vi "PDCGetAllStates.vi"(8 "error in (no error)":errorcluster, 10 "PDCLists":T5, 11 "PDCAllStates in":T1={"DeviceNo"=0, "ChildNo"=1, "ColorType"=enum."MONO", "BitDepth"=0, "Resolution"={"Width"=0, "Height"=0}, "RecordRate"=0, "ShutterSpeed"=0, "TriggerMode"=0, "Display"=enum."LiveStop", "PDCRecordStatus"=enum."Live", "PlayFrames"=FALSE, "Start Frame"=0, "Current Frame"=0, "End Frame"=0, "RefImage8bit"=[], "RefImage16bit"=[], "Auto Trigger"=FALSE, "PDCSettings"={"Interface"=enum."Gigabit-Ethernet", "AutoSearch"=FALSE, "IP - AutoSearch"=[], "IP - Direct"=[], "Simulate"=FALSE}}) -> (0 "error out":errorcluster, 2 "PDC Setup":T6={"Color Type"=enum."MONO", "Bit Depth"=0, "Resolution"=0, "Record Rate"=0, "Shutter Speed"=0, "Trigger Mode"=0, "Display"=enum."LiveStop"} {"Trigger Mode" items=["START", "CENTER", "END", "MANUAL", "RANDOM", "RANDOM_RESET", "RANDOM_CENTER", "RANDOM_MANUAL", "START", "START"]; "Shutter Speed" items=["1/42772 sec", "1/44444 sec", "1/47058 sec", "1/50000 sec", "1/53333 sec", "1/57142 sec", "1/61538 sec", "1/66666 sec", "1/72727 sec", "1/80000 sec", "1/88888 sec", "1/100000 sec", "1/114285 sec", "1/133333 sec", "1/160000 sec", "1/200000 sec", "1/266666 sec", "1/400000 sec", "1/800000 sec", "1/996923 sec", "1/1246154 sec", "1/1661538 sec", "1/2700000 sec", "1/3410526 sec"]; "Resolution" items=["768 X 416", "896 X 368", "768 X 328", "768 X 272", "640 X 256", "512 X 512", "512 X 272", "512 X 256", "384 X 264", "256 X 256", "256 X 152", "256 X 128", "256 X 80", "128 X 128", "128 X 48", "128 X 40", "128 X 16", "128 X 8"]; "Record Rate" items=["50 fps", "60 fps", "125 fps", "250 fps", "500 fps", "1000 fps", "2000 fps", "3000 fps", "4000 fps", "5000 fps", "6000 fps", "7200 fps", "8000 fps", "9000 fps", "10000 fps", "12500 fps", "13500 fps", "20000 fps", "30000 fps", "40000 fps", "50000 fps", "60000 fps", "72000 fps", "81000 fps", "100000 fps", "200000 fps", "300000 fps", "480000 fps", "540000 fps", "675000 fps", "900000 fps", "1080000 fps"]}, 3 "PDCAllStates out":T1={"DeviceNo"=0, "ChildNo"=1, "ColorType"=enum."MONO", "BitDepth"=0, "Resolution"={"Width"=0, "Height"=0}, "RecordRate"=0, "ShutterSpeed"=0, "TriggerMode"=0, "Display"=enum."LiveStop", "PDCRecordStatus"=enum."Live", "PlayFrames"=FALSE, "Start Frame"=0, "Current Frame"=0, "End Frame"=0, "RefImage8bit"=[], "RefImage16bit"=[], "Auto Trigger"=FALSE, "PDCSettings"={"Interface"=enum."Gigabit-Ethernet", "AutoSearch"=FALSE, "IP - AutoSearch"=[], "IP - Direct"=[], "Simulate"=FALSE}})   [LabVIEW 2015]
uses:
  TypeDefs/PDCSetup.ctl
  TypeDefs/PDCDisplay.ctl
  TypeDefs/PDCAllStates.ctl
  TypeDefs/PDCRecordStatus.ctl
  TypeDefs/PDCSettings.ctl
  TypeDefs/PDCLists.ctl
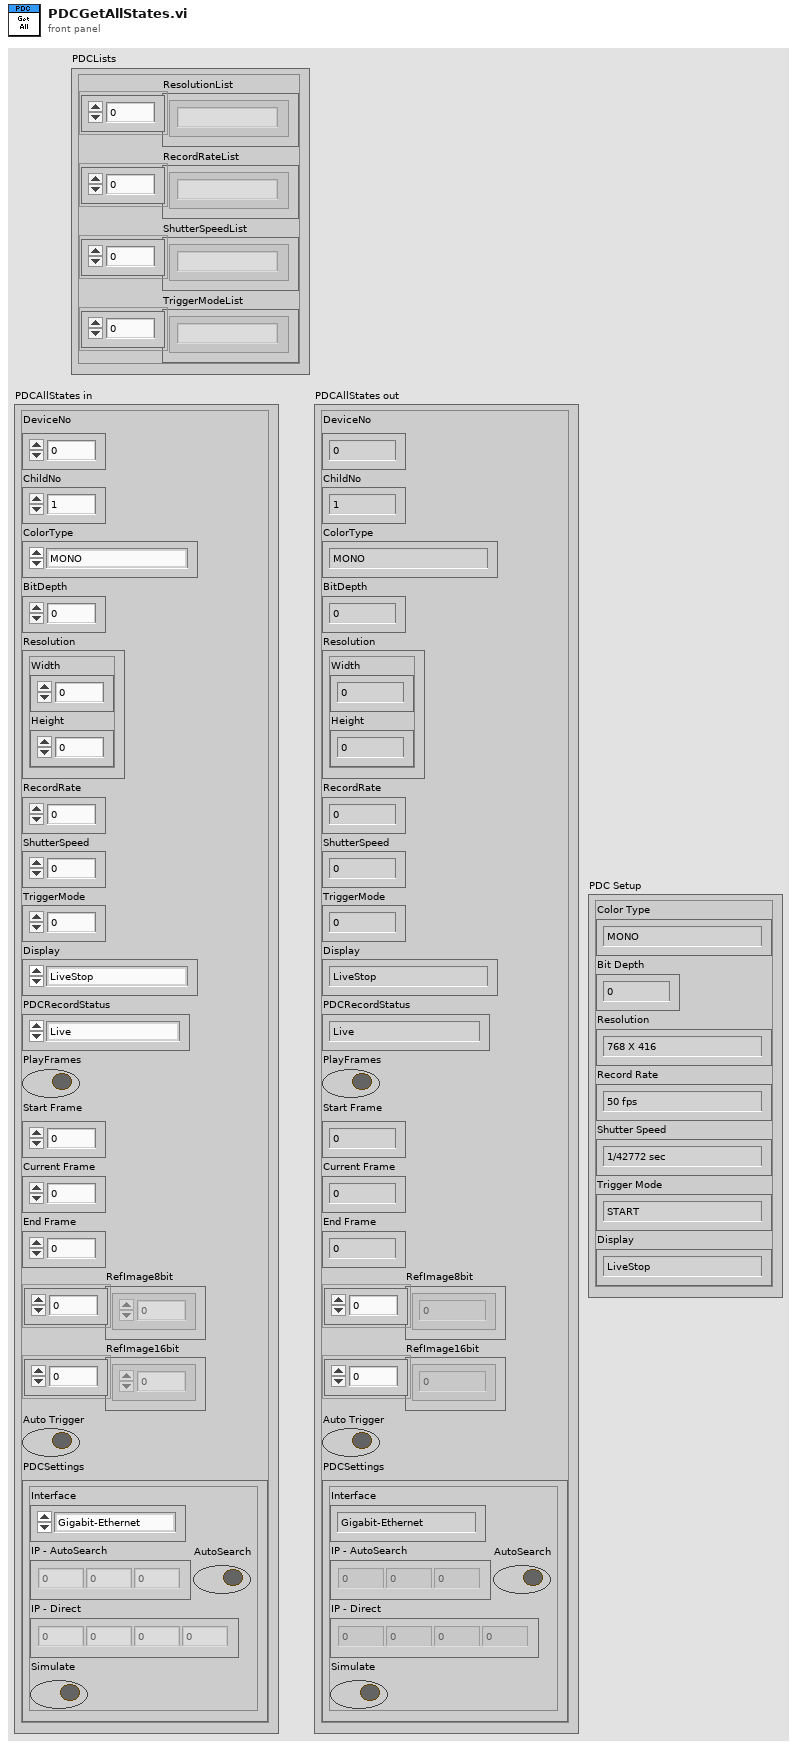
[diagram p1: front panel]
types:
  T1 = typedef "PDCAllStates.ctl" = cluster{"DeviceNo":u32, "ChildNo":u32, "ColorType":enum16{"MONO", "COLOR"}, "BitDepth":i8, "Resolution":cluster{"Width":u32, "Height":u32}, "RecordRate":u32, "ShutterSpeed":u32, "TriggerMode":u32, "Display":T2, "PDCRecordStatus":T3, "PlayFrames":bool, "Start Frame":i32, "Current Frame":i32, "End Frame":i32, "RefImage8bit":u8[], "RefImage16bit":u16[], "Auto Trigger":bool, "PDCSettings":T4}
  T2 = typedef "PDCDisplay.ctl" = enum16{"Live", "Memory", "LiveStop"}
  T3 = typedef "PDCRecordStatus.ctl" = enum16{"Live", "Endless", "Recording"}
  T4 = typedef "PDCSettings.ctl" = cluster{"Interface":enum16{"Gigabit-Ethernet", "IEEE1394a", "Photron Optical", "PCI/PCI Express"}, "AutoSearch":bool, "IP - AutoSearch":u32[], "IP - Direct":u32[], "Simulate":bool}
  T5 = typedef "PDCLists.ctl" = cluster{"ResolutionList":string[], "RecordRateList":string[], "ShutterSpeedList":string[], "TriggerModeList":string[]}
  T6 = typedef "PDCSetup.ctl" = cluster{"Color Type":enum16{"MONO", "COLOR"}, "Bit Depth":i8, "Resolution":u16, "Record Rate":u16, "Shutter Speed":u16, "Trigger Mode":u16, "Display":T2}
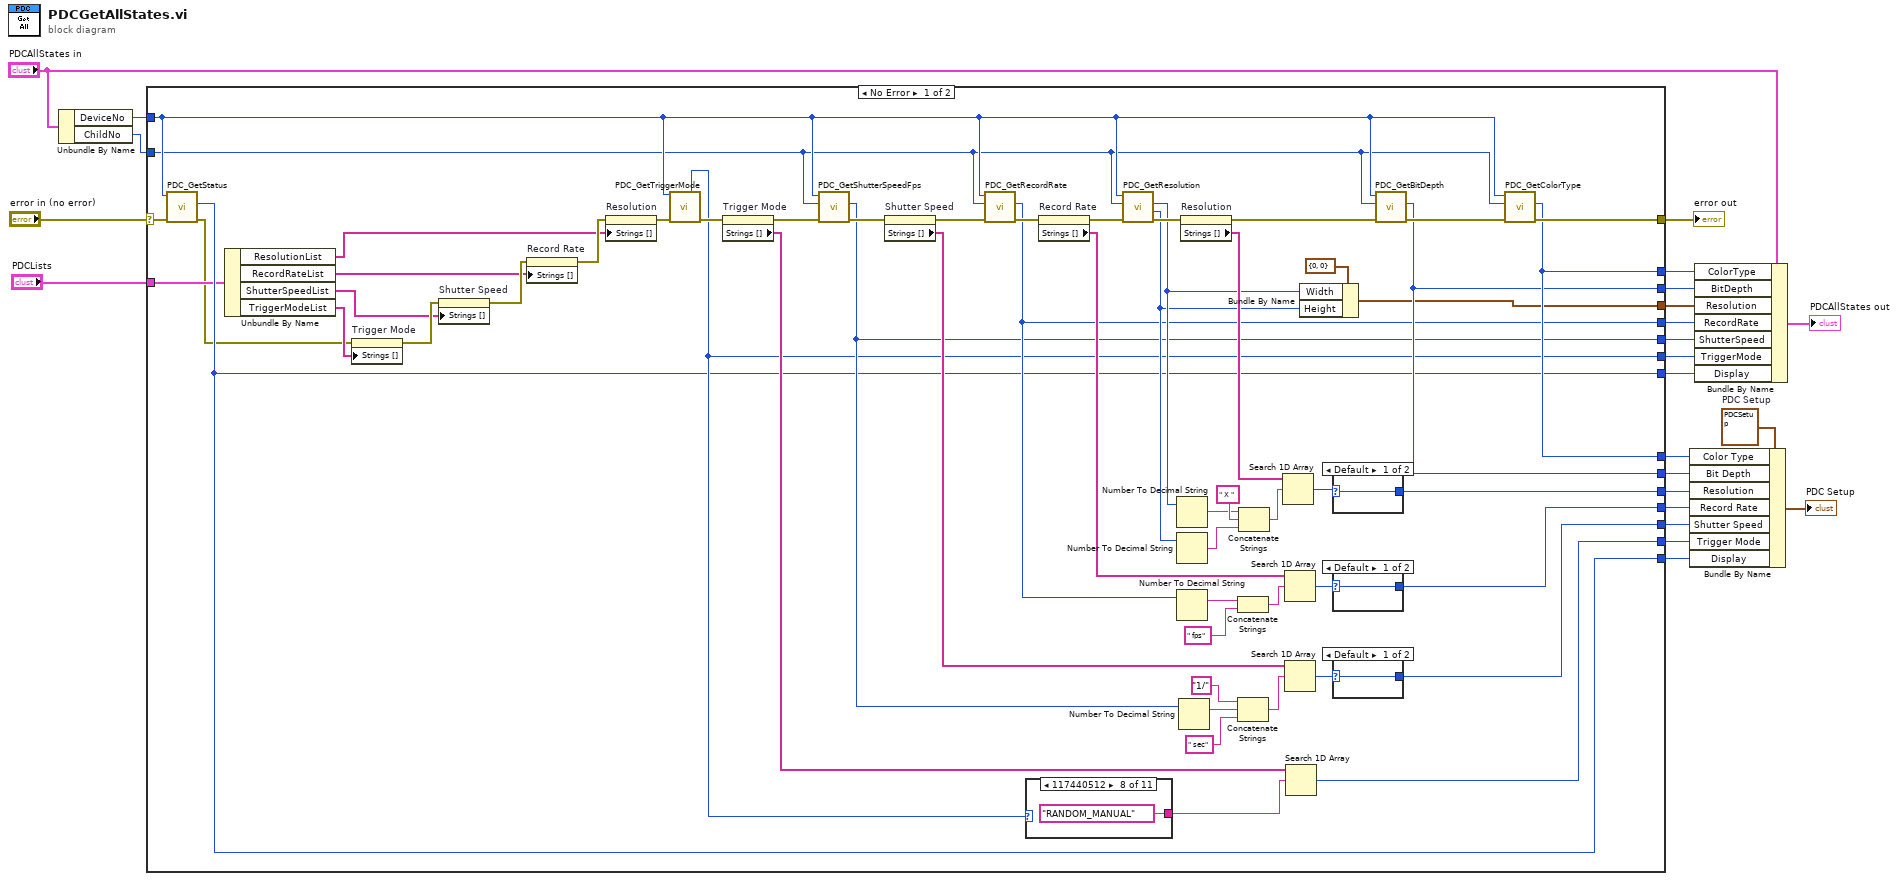
[diagram p0: block diagram]
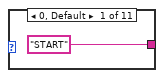
[diagram p2: hidden frame]
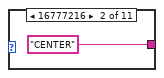
[diagram p3: hidden frame]
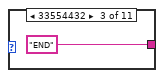
[diagram p4: hidden frame]
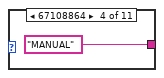
[diagram p5: hidden frame]
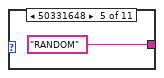
[diagram p6: hidden frame]
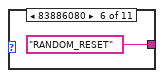
[diagram p7: hidden frame]
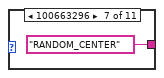
[diagram p8: hidden frame]
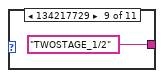
[diagram p9: hidden frame]
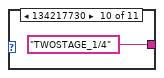
[diagram p10: hidden frame]
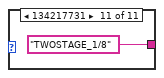
[diagram p11: hidden frame]
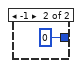
[diagram p12: hidden frame]
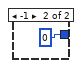
[diagram p13: hidden frame]
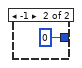
[diagram p14: hidden frame]
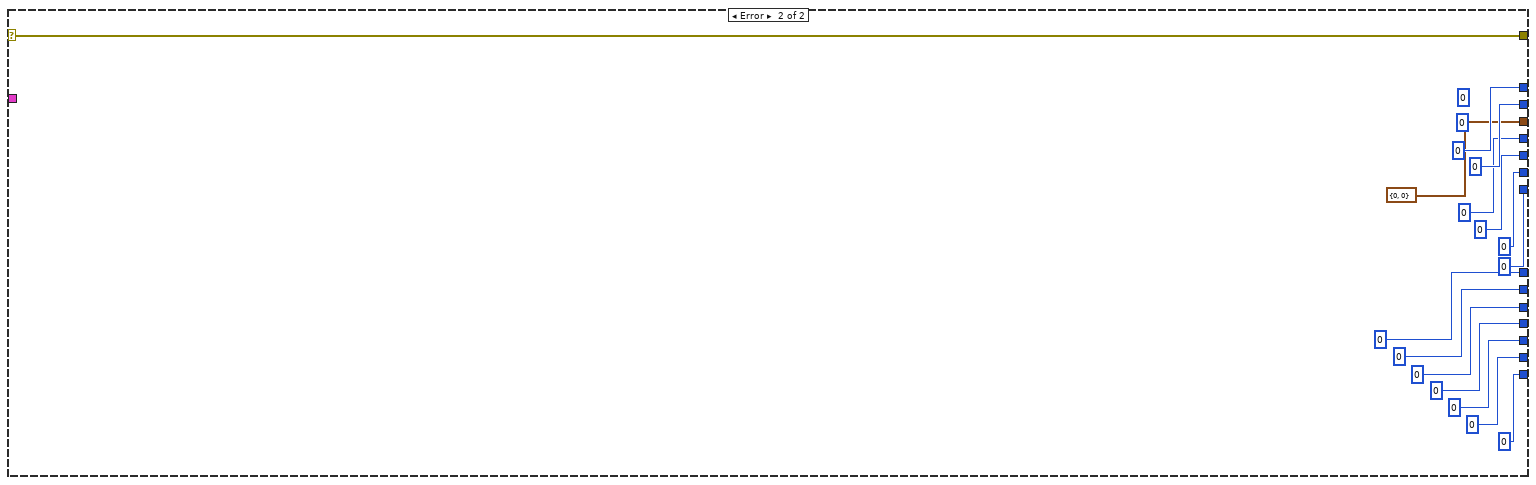
[diagram p15: hidden frame]
diagram:
  w21 = T6 {"Color Type"=enum."MONO", "Bit Depth"=0, "Resolution"=0, "Record Rate"=0, "Shutter Speed"=0, "Trigger Mode"=0, "Display"=enum."LiveStop"}  # PDC Setup
  n1 = Unbundle By Name("PDCAllStates in") -> ("DeviceNo"=w3:u32, "ChildNo"=w2:u32)
  n2 = case shown="No Error" "error in (no error)" {
    selector: "error in (no error)" -> [w34 w111]
    tunnel: [w78 w111] -> w23
    tunnel: [w42 i8 0 ("Mode")] -> w19
    tunnel: [w41 i8 0 ("Depth")] -> w18
    tunnel: [w68 0 ("index of element")] -> w17
    tunnel: [w61 0 ("index of element")] -> w16
    tunnel: [w55 0 ("index of element")] -> w15
    tunnel: [w43 0 ("index of element")] -> w14
    tunnel: [w42 i8 0 ("Mode")] -> w13
    tunnel: [w41 i8 0 ("Depth")] -> w12
    tunnel: [w40 cluster{"Width":u32, "Height":u32} {"Width"=0, "Height"=0} ("Resolution")] -> w4
    tunnel: [w37 u32 0 ("Rate")] -> w11
    tunnel: [w36 u32 0 ("Fps")] -> w10
    tunnel: [w35 u32 0 ("Mode")] -> w9
    tunnel: [w33 u32 0 ("Status")] -> w7
    tunnel: [w33 u32 0 ("Status")] -> w6
    tunnel: "PDCLists" -> [w32 _]
    tunnel: w3 -> [w25 _]
    tunnel: w2 -> [w24 _]
    frame No Error {
      n3 = call "PDC_GetStatus.vi"("error in (no error)"=w34, "DeviceNo"=w25) -> ("error out"=w27:errorcluster, "Status"=w33:u32)  [unwired: 6 in, 2 out]
      n4 = Unbundle By Name(w32) -> ("ResolutionList"=w31:string[], "RecordRateList"=w30:string[], "ShutterSpeedList"=w28:string[], "TriggerModeList"=w29:string[])
      n5 = property on="Trigger Mode" class="Ring (strict)"(error in=w27, "Strings []"=w29) -> (error out=w76:errorcluster)  [unwired: 1 in, 1 out]
      n6 = property on="Shutter Speed" class="Ring (strict)"(error in=w76, "Strings []"=w28) -> (error out=w75:errorcluster)  [unwired: 1 in, 1 out]
      n7 = property on="Record Rate" class="Ring (strict)"(error in=w75, "Strings []"=w30) -> (error out=w74:errorcluster)  [unwired: 1 in, 1 out]
      n8 = property on="Resolution" class="Ring (strict)"(error in=w74, "Strings []"=w31) -> (error out=w54:errorcluster)  [unwired: 1 in, 1 out]
      n9 = call "PDC_GetTriggerMode.vi"("DeviceNo"=w25, "error in (no error)"=w54) -> ("Mode"=w35:u32, "error out"=w47:errorcluster)  [unwired: 7 in, 5 out]
      n10 = property on="Trigger Mode" class="Ring (strict)"(error in=w47) -> (error out=w46:errorcluster, "Strings []"=w45:string[])  [unwired: 1 in, 1 out]
      n11 = call "PDC_GetShutterSpeedFps.vi"("error in (no error)"=w46, "ChildNo"=w24, "DeviceNo"=w25) -> ("error out"=w50:errorcluster, "Fps"=w36:u32)  [unwired: 5 in, 2 out]
      n12 = property on="Shutter Speed" class="Ring (strict)"(error in=w50) -> (error out=w49:errorcluster, "Strings []"=w48:string[])  [unwired: 1 in, 1 out]
      n13 = call "PDC_GetRecordRate.vi"("error in (no error)"=w49, "ChildNo"=w24, "DeviceNo"=w25) -> ("error out"=w53:errorcluster, "Rate"=w37:u32)  [unwired: 5 in, 2 out]
      n14 = case shown="117440512" w35 {
        tunnel: ["START" "CENTER" "END" "MANUAL" "RANDOM" "RANDOM_RESET" "RANDOM_CENTER" "RANDOM_MANUAL" "TWOSTAGE_1/2" "TWOSTAGE_1/4" "TWOSTAGE_1/8"] -> w44
        frame 0, Default {
        }
        frame 16777216 {
        }
        frame 33554432 {
        }
        frame 67108864 {
        }
        frame 50331648 {
        }
        frame 83886080 {
        }
        frame 100663296 {
        }
        frame 117440512 {
        }
        frame 134217729 {
        }
        frame 134217730 {
        }
        frame 134217731 {
        }
      }
      n15 = property on="Record Rate" class="Ring (strict)"(error in=w53) -> (error out=w52:errorcluster, "Strings []"=w51:string[])  [unwired: 1 in, 1 out]
      n16 = call "PDC_GetResolution.vi"("error in (no error)"=w52, "ChildNo"=w24, "DeviceNo"=w25) -> ("error out"=w79:errorcluster, "Height"=w38:u32, "Width"=w39:u32)  [unwired: 4 in, 2 out]
      n17 = Number To Decimal String(number=w39) -> (decimal integer string=w71:string)  [unwired: 1 out]
      n18 = Number To Decimal String(number=w38) -> (decimal integer string=w70:string)  [unwired: 1 out]
      n19 = Number To Decimal String(number=w37) -> (decimal integer string=w64:string)  [unwired: 1 out]
      n20 = Number To Decimal String(number=w36) -> (decimal integer string=w60:string)  [unwired: 1 out]
      n21 = property on="Resolution" class="Ring (strict)"(error in=w79) -> (error out=w67:errorcluster, "Strings []"=w66:string[])  [unwired: 1 in, 1 out]
      n22 = Concatenate Strings(w64, " fps") -> (w65:string)
      n23 = Concatenate Strings("1/", w60, " sec") -> (w58:string)
      n24 = Concatenate Strings(w71, " X ", w70) -> (w73:string)
      n25 = Search 1D Array(1D array=w66, element=w73) -> (index of element=w69:i32)  [unwired: 1 in]
      n26 = Search 1D Array(1D array=w51, element=w65) -> (index of element=w62:i32)  [unwired: 1 out]
      n27 = Search 1D Array(1D array=w48, element=w58) -> (index of element=w56:i32)  [unwired: 1 out]
      n28 = Search 1D Array(1D array=w45, element=w44) -> (index of element=w43:i32)  [unwired: 1 out]
      n29 = Bundle By Name(cluster=cluster{"Width":u32, "Height":u32} {"Width"=0, "Height"=0} ("Resolution"), "Width"=w39, "Height"=w38) -> (w40:cluster{"Width":u32, "Height":u32})
      n30 = case shown="Default" w69 {
        selector: w69 -> [w95 _]
        tunnel: [w95 0 ("index of element")] -> w68
        frame Default {
        }
        frame -1 {
        }
      }
      n31 = case shown="Default" w62 {
        selector: w62 -> [w93 _]
        tunnel: [w93 0 ("index of element")] -> w61
        frame Default {
        }
        frame -1 {
        }
      }
      n32 = case shown="Default" w56 {
        selector: w56 -> [w91 _]
        tunnel: [w91 0 ("index of element")] -> w55
        frame Default {
        }
        frame -1 {
        }
      }
      n33 = call "PDC_GetBitDepth.vi"("error in (no error)"=w67, "ChildNo"=w24, "DeviceNo"=w25) -> ("error out"=w77:errorcluster, "Depth"=w41:i8)  [unwired: 5 in, 2 out]
      n34 = call "PDC_GetColorType.vi"("error in (no error)"=w77, "ChildNo"=w24, "DeviceNo"=w25) -> ("error out"=w78:errorcluster, "Mode"=w42:i8)  [unwired: 5 in, 2 out]
    }
    frame Error {
      (unwired) u32 0 ("ChildNo")
      (unwired) u32 0 ("DeviceNo")
    }
  }
  "error out" <- w23
  n35 = Bundle By Name(cluster=w21, "Color Type"=w19, "Bit Depth"=w18, "Resolution"=w17, "Record Rate"=w16, "Shutter Speed"=w15, "Trigger Mode"=w14, "Display"=w6) -> (→"PDC Setup":T6)
  n36 = Bundle By Name(cluster="PDCAllStates in", "ColorType"=w13, "BitDepth"=w12, "Resolution"=w4, "RecordRate"=w11, "ShutterSpeed"=w10, "TriggerMode"=w9, "Display"=w7) -> (→"PDCAllStates out":T1)
